vi "Error Message Icons.vi"() -> (2 "open":i32=15, 3 "closed":i32=14)   [LabVIEW 2021, in "MeasurementClient Editor.lvlib"]
uses:
  MeasurementClient Editor.lvlib
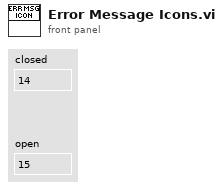
[diagram p1: front panel]
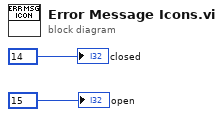
[diagram p0: block diagram]
diagram:
  "closed" <- 14
  "open" <- 15
